vi "ReadDeviceJSONList.vi"(8 "error in":errorcluster, 11 "JSON":string="{}") -> (0 "error out":errorcluster, 3 "table of devices":string[](array[string]))   [LabVIEW 2023, in "GenericDevice.lvclass"]
doc: "Parses the returned devies into a string array."
uses:
  GenericDevice.lvclass
  70255800-8428-4597-ad6a-1f50491d66f4.vi
  <vilib>/JDP Science/JSONtext/Find Item.vi
  <vilib>/JDP Science/JSONtext/Next JSON Value.vi
  <vilib>/JDP Science/JSONtext/String Subset.vi
  <vilib>/JDP Science/JSONtext/Parsing/Advance past next JSON Value (inlined COPY).vi
  <vilib>/JDP Science/JSONtext/Parsing/Advance past whitespace.vi
  <vilib>/JDP Science/JSONtext/Parsing/Advance past String.vi
  <vilib>/JDP Science/JSONtext/Parsing/Advance past Number.vi
  <vilib>/JDP Science/JSONtext/Parsing/Advance past Line Ending.vi
  <vilib>/JDP Science/JSONtext/Parsing/Parse Full Path or Item Name.vi
  <vilib>/JDP Science/JSONtext/Parsing/Advance past Array.vi
  <vilib>/JDP Science/JSONtext/Parsing/Advance past Object.vi
  <vilib>/JDP Science/JSONtext/support/Error Cluster From Code.vi
  <vilib>/JDP Science/JSONtext/Offset/Find Item Locations by Path.vi
  <vilib>/JDP Science/JSONtext/JSON text to Variant.vi
  <vilib>/JDP Science/JSONtext/LVClass Serializer/JSONtext LVClass Serializer.lvclass
panel:
  # "Connector Pane"
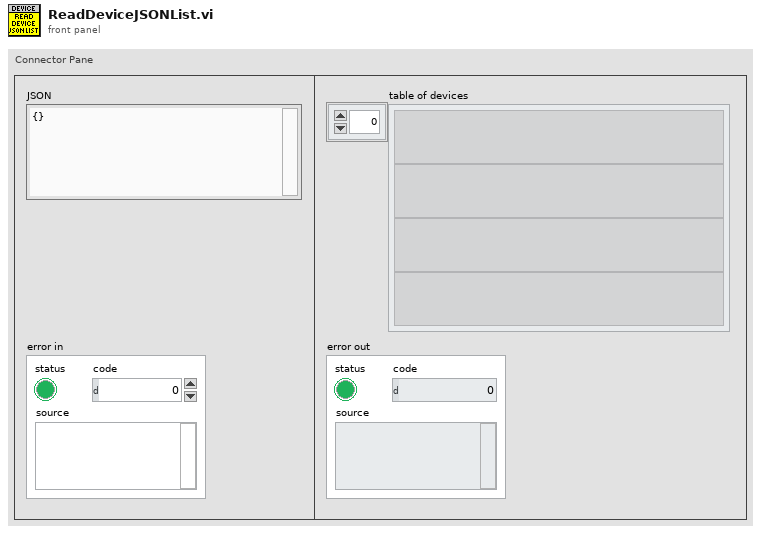
[diagram p1: front panel]
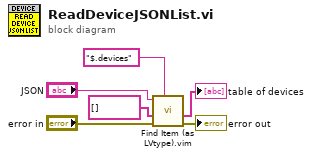
[diagram p0: block diagram]
diagram:
  n1 = call "Find Item (as LVtype).vim"("$Path or Item Name"="$.devices" ("Label (VI Title)"), "error in (no error)"="error in", "Data Type and Default Value"=string[] [], "JSON"="JSON") -> ("error out"=→"error out":errorcluster, "Data"=→"table of devices":string[])  [unwired: 4 in, 2 out]
